vi "GroupOnlyNormalHeavyImplefixaddtimeaddLED.vi"() -> ()   [LabVIEW 2021]
uses:
  ControlforGroupOnlyNormalHeavyImple.ctl
  Control 1.ctl
panel:
  out "speed of train":string
  out "Traffic":string
  out "Traffic condition":string
  out "train":string
  out "Number of Car 2":dbl
  out "Stop of traffic":i32
  out "Wait Time for Train":i32
  out "Number of Car":dbl
  in  "stop":bool
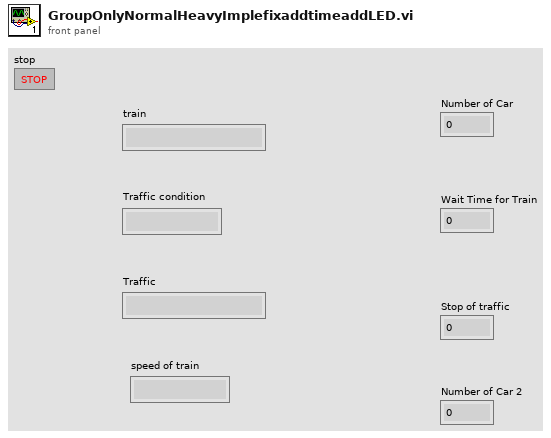
[diagram p1: front panel]
types:
  T1 = typedef "Control 1.ctl" = enum16{"wait", "Down", "Up"}
  T2 = typedef "ControlforGroupOnlyNormalHeavyImple.ctl" = enum16{"Normal", "Heavy", "AfterHeavy"}
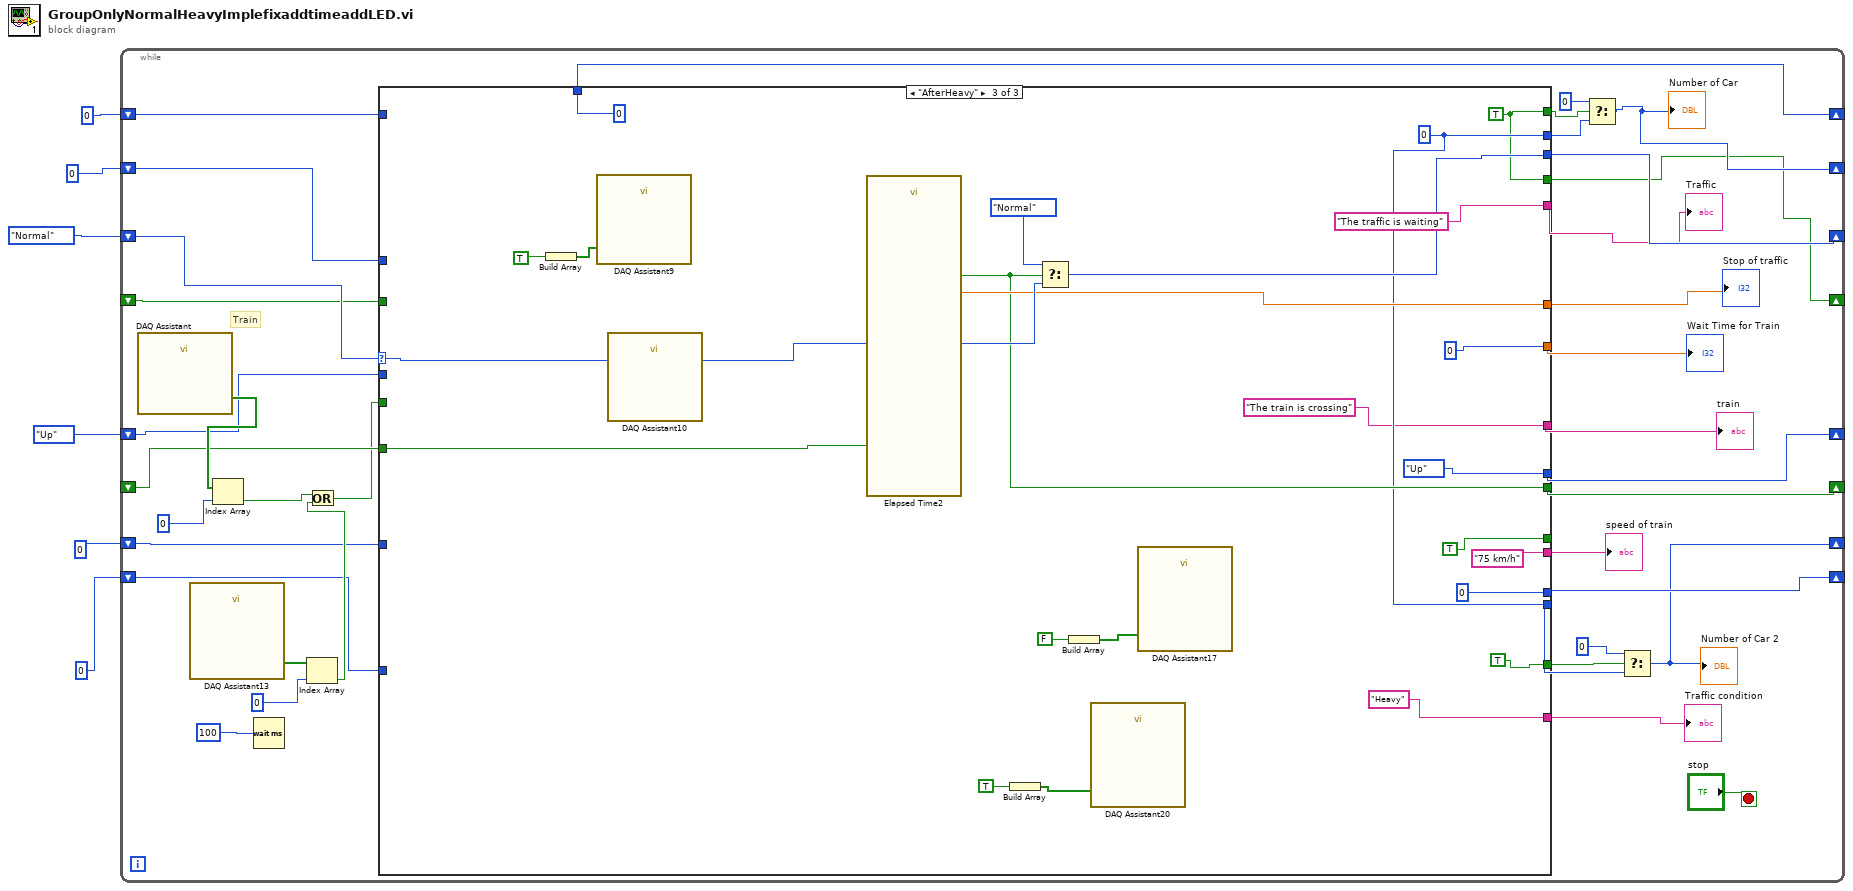
[diagram p0: block diagram]
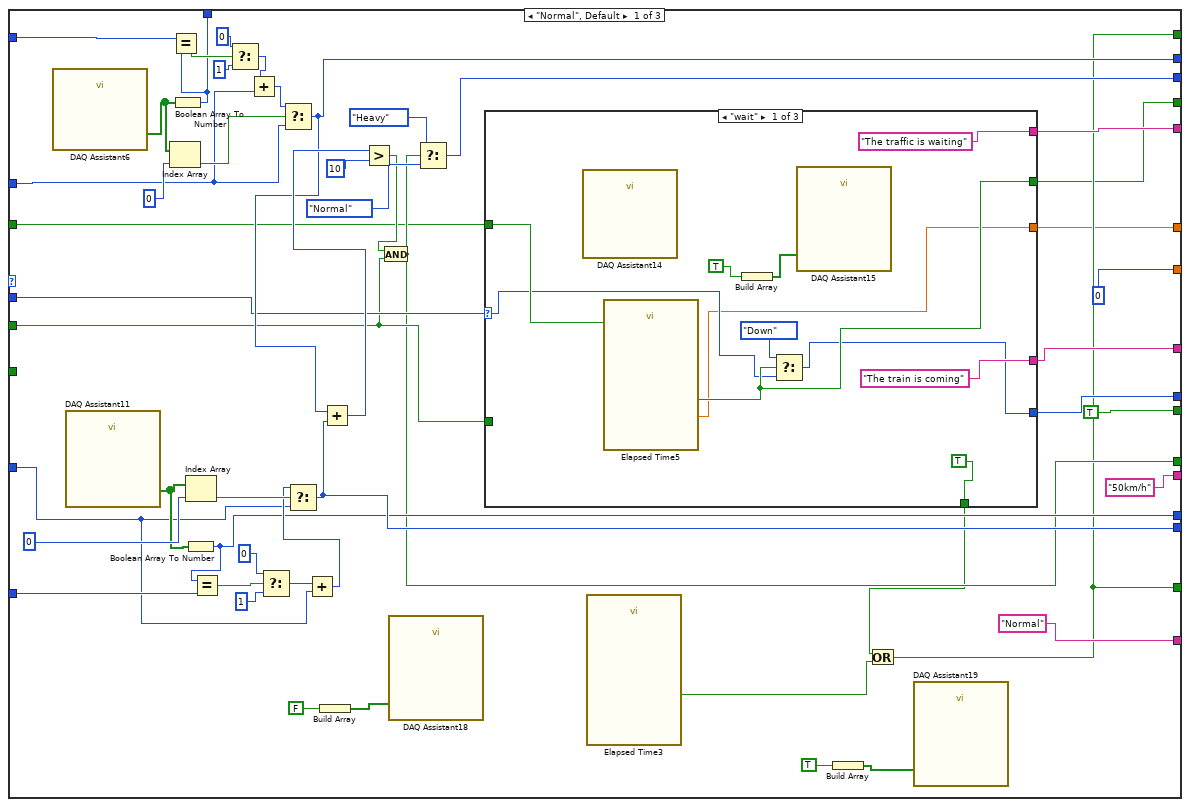
[diagram p2: hidden frame]
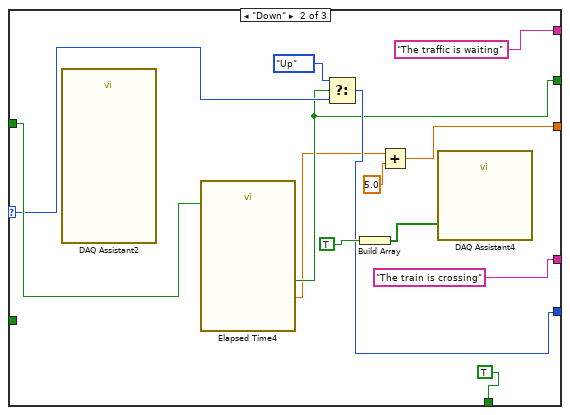
[diagram p3: hidden frame]
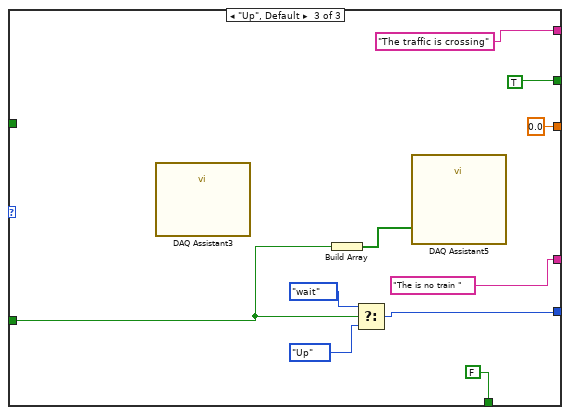
[diagram p4: hidden frame]
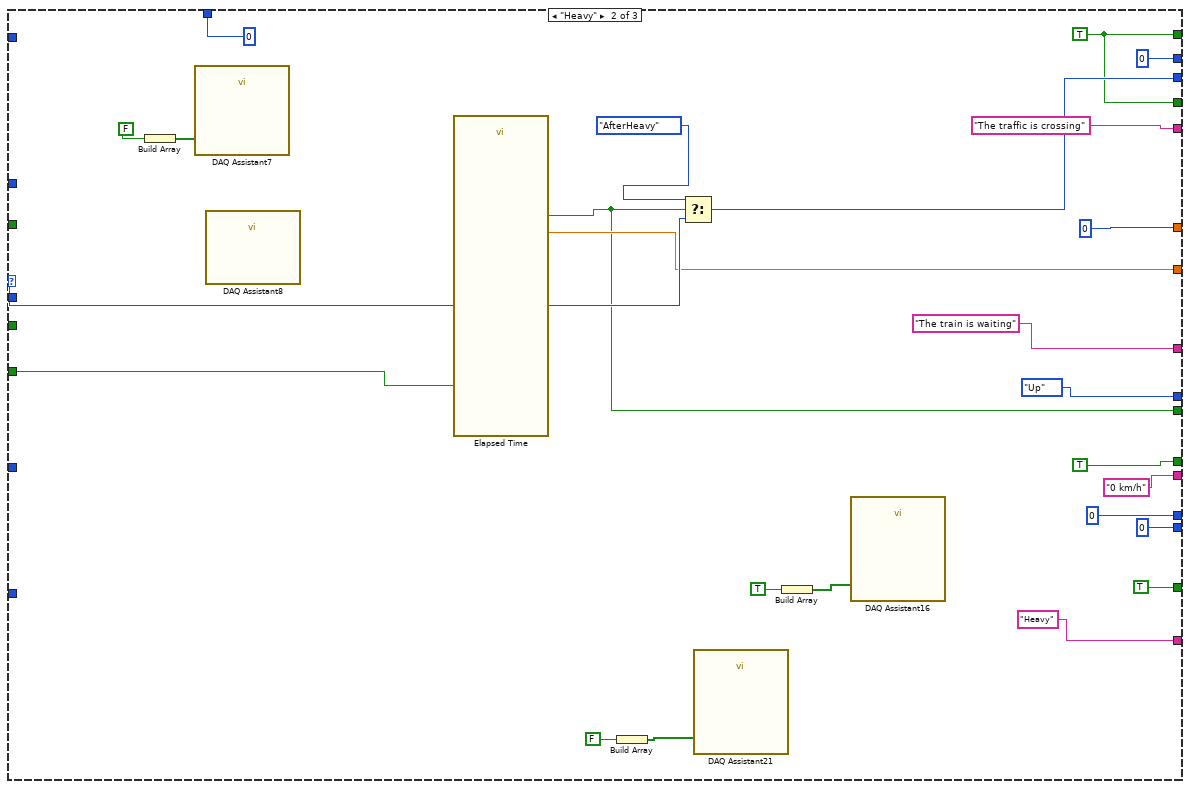
[diagram p5: hidden frame]
diagram:
  n1 = while {
    shift-right: [w41] -> _
    shift-left: ControlforGroupOnlyNormalHeavyImple."Normal" -> [w40]
    shift-right: [w14] -> _
    shift-left: 0 -> [w29]
    shift-right: [w36] -> _
    shift-left: _ -> [w35]
    shift-right: [w18] -> _
    shift-left: 0 -> [w28]
    shift-right: [w16] -> _
    shift-left: 0 ("index") -> [w27]
    shift-right: [w25] -> _
    shift-left: Control_1."Up" -> [w26]
    shift-right: [w23] -> _
    shift-left: 0 ("index") -> [w24]
    shift-right: [w12] -> _
    shift-left: _ -> [w11]
    stop <- "stop" stop-if-true
    # "Train"
    n2 = call "DAQ Assistant"() -> ("data"=w42:bool[])  [unwired: 17 in, 2 out]
    n3 = call "DAQ Assistant13"() -> ("data"=w33:bool[])  [unwired: 17 in, 2 out]
    n4 = Index Array(array=w42, index=0) -> (element=w32:bool)
    n5 = Wait (ms)(milliseconds to wait=100) -> ()  [unwired: 1 out]
    n6 = Index Array(array=w33, index=0) -> (element=w31:bool)
    n7 = Or(x=w32, y=w31) -> (x .or. y?=w21:bool)
    n8 = case shown="\"AfterHeavy\"" w40 {
      selector: w40 -> [_ w148 w173]
      tunnel: w21 -> [w56 _ _]
      tunnel: [w90 w149 w172] -> w41
      tunnel: w29 -> [w69 _ _]
      tunnel: [w84 0 w167] -> w15
      tunnel: [w51 0 w170] -> w38
      tunnel: [0 w146 0] -> w37
      tunnel: [TRUE w145 w169] -> w36
      tunnel: w35 -> [_ w144 w168]
      tunnel: w28 -> [w61 _ _]
      tunnel: [w85 0 w167] -> w19
      tunnel: w27 -> [w82 _ _]
      tunnel: [w77 u32 0 ("index") u32 0 ("index")] -> w16
      tunnel: w26 -> [w76 _ _]
      tunnel: [w75 Control_1."Up" Control_1."Up"] -> w25
      tunnel: w24 -> [w62 _ _]
      tunnel: [w63 u32 0 u32 0] -> w23
      tunnel: ["Normal" "Heavy" "Heavy"] -> w22
      tunnel: [w59 "The train is waiting" "The train is crossing"] -> w9
      tunnel: [w58 "The traffic is crossing" "The traffic is waiting"] -> w10
      tunnel: [w55 TRUE TRUE] -> _
      tunnel: [w52 TRUE TRUE] -> w8
      tunnel: [w52 w131 w156] -> w13
      tunnel: [w50 w131 w156] -> w12
      tunnel: w11 -> [w49 _ _]
      tunnel: ["50km/h" "0 km/h" "75 km/h"] -> w7
      frame "Normal", Default {
        n9 = call "DAQ Assistant6"() -> ("data"=w80:bool[])  [unwired: 17 in, 2 out]
        n10 = call "DAQ Assistant11"() -> ("data"=w74:bool[])  [unwired: 17 in, 2 out]
        n11 = Index Array(array=w80, index=0) -> (element=w81:bool)
        n12 = Boolean Array To Number(Boolean array=w80) -> (number=w77:u32)
        n13 = Equal?(x=w82, y=w77) -> (x = y?=w79:bool)
        n14 = Index Array(array=w74, index=0) -> (element=w65:bool)
        n15 = Boolean Array To Number(Boolean array=w74) -> (number=w63:u32)
        n16 = Equal?(x=w63, y=w62) -> (x = y?=w73:bool)
        n17 = Select(t=0, s=w79, f=1) -> (s? t:f=w70:i32)
        n18 = Add(x=w70, y=w69) -> (x+y=w68:i32)
        n19 = Select(t=0, s=w73, f=1) -> (s? t:f=w66:i32)
        n20 = Select(t=w68, s=w81, f=w69) -> (s? t:f=w84:i32)
        n21 = Add(x=w66, y=w61) -> (x+y=w64:i32)
        n22 = Select(t=w64, s=w65, f=w61) -> (s? t:f=w85:i32)
        n23 = Build Array(FALSE) -> (w48:bool[])
        n24 = Add(x=w84, y=w85) -> (x+y=w86:i32)
        n25 = Greater?(x=w86, y=10) -> (0:w57:bool)
        n26 = And(x=w57, y=w56) -> (x .and. y?=w55:bool)
        n27 = call "DAQ Assistant18"("data"=w48) -> ()  [unwired: 17 in, 2 out]
        n28 = Select(t=ControlforGroupOnlyNormalHeavyImple."Heavy", s=w55, f=ControlforGroupOnlyNormalHeavyImple."Normal") -> (s? t:f=w90:T2)
        n29 = case shown="\"wait\"" w76 {
          selector: w76 -> [w96 w110 _]
          tunnel: w56 -> [_ _ w120]
          tunnel: [w98 w109 w126] -> w75
          tunnel: ["The train is coming" "The train is crossing" "The is no train "] -> w59
          tunnel: ["The traffic is waiting" "The traffic is waiting" "The traffic is crossing"] -> w58
          tunnel: [TRUE TRUE FALSE] -> w53
          tunnel: [w95 w105 0.0 ("Elapsed Time (s)")] -> w51
          tunnel: [w99 w108 TRUE] -> w50
          tunnel: w49 -> [w100 w112 _]
          frame "wait" {
            n30 = call "DAQ Assistant14"() -> ()  [unwired: 18 in, 2 out]
            n31 = call "Elapsed Time5"("Reset"=w100) -> ("Elapsed Time (s)"=w95:dbl, "Time has Elapsed"=w99:bool)  [unwired: 11 in, 6 out]
            n32 = Build Array(TRUE) -> (w104:bool[])
            n33 = Select(t=Control_1."Down", s=w99, f=w96) -> (s? t:f=w98:T1)
            n34 = call "DAQ Assistant15"("data"=w104) -> ()  [unwired: 17 in, 2 out]
          }
          frame "Down" {
            n35 = call "DAQ Assistant2"() -> ()  [unwired: 18 in, 2 out]
            n36 = call "Elapsed Time4"("Reset"=w112) -> ("Elapsed Time (s)"=w106:dbl, "Time has Elapsed"=w108:bool)  [unwired: 11 in, 6 out]
            n37 = Select(t=Control_1."Up", s=w108, f=w110) -> (s? t:f=w109:T1)
            n38 = Build Array(TRUE) -> (w117:bool[])
            n39 = Add(x=w106, y=5.0) -> (x+y=w105:dbl)
            n40 = call "DAQ Assistant4"("data"=w117) -> ()  [unwired: 17 in, 2 out]
          }
          frame "Up", Default {
            n41 = call "DAQ Assistant3"() -> ()  [unwired: 18 in, 2 out]
            n42 = Build Array(w120) -> (w127:bool[])
            n43 = Select(t=Control_1."wait", s=w120, f=Control_1."Up") -> (s? t:f=w126:T1)
            n44 = call "DAQ Assistant5"("data"=w127) -> ()  [unwired: 17 in, 2 out]
          }
        }
        n45 = call "Elapsed Time3"() -> ("Time has Elapsed"=w54:bool)  [unwired: 12 in, 7 out]
        n46 = Build Array(TRUE) -> (w44:bool[])
        n47 = Or(x=w53, y=w54) -> (x .or. y?=w52:bool)
        n48 = call "DAQ Assistant19"("data"=w44) -> ()  [unwired: 17 in, 2 out]
      }
      frame "Heavy" {
        w131 = TRUE
        n49 = Build Array(FALSE) -> (w151:bool[])
        n50 = call "DAQ Assistant7"("data"=w151) -> ()  [unwired: 17 in, 2 out]
        n51 = call "DAQ Assistant8"() -> ()  [unwired: 18 in, 2 out]
        n52 = call "Elapsed Time"("Reset"=w144) -> ("Elapsed Time (s)"=w146:dbl, "Time has Elapsed"=w145:bool)  [unwired: 11 in, 6 out]
        n53 = Build Array(FALSE) -> (w128:bool[])
        n54 = Select(t=ControlforGroupOnlyNormalHeavyImple."AfterHeavy", s=w145, f=w148) -> (s? t:f=w149:T2)
        n55 = call "DAQ Assistant21"("data"=w128) -> ()  [unwired: 17 in, 2 out]
        n56 = Build Array(TRUE) -> (w137:bool[])
        n57 = call "DAQ Assistant16"("data"=w137) -> ()  [unwired: 17 in, 2 out]
      }
      frame "AfterHeavy" {
        w156 = TRUE
        w167 = 0
        n58 = Build Array(TRUE) -> (w175:bool[])
        n59 = call "DAQ Assistant9"("data"=w175) -> ()  [unwired: 17 in, 2 out]
        n60 = call "DAQ Assistant10"() -> ()  [unwired: 18 in, 2 out]
        n61 = call "Elapsed Time2"("Reset"=w168) -> ("Elapsed Time (s)"=w170:dbl, "Time has Elapsed"=w169:bool)  [unwired: 11 in, 6 out]
        n62 = Build Array(TRUE) -> (w154:bool[])
        n63 = Select(t=ControlforGroupOnlyNormalHeavyImple."Normal", s=w169, f=w173) -> (s? t:f=w172:T2)
        n64 = Build Array(FALSE) -> (w161:bool[])
        n65 = call "DAQ Assistant20"("data"=w154) -> ()  [unwired: 17 in, 2 out]
        n66 = call "DAQ Assistant17"("data"=w161) -> ()  [unwired: 17 in, 2 out]
      }
    }
    "Wait Time for Train" <- w37
    "Stop of traffic" <- w38
    "Traffic condition" <- w22
    "train" <- w9
    "Traffic" <- w10
    "speed of train" <- w7
    n67 = Select(t=0, s=w13, f=w15) -> (s? t:f=w14:i32)
    "Number of Car" <- w14
    n68 = Select(t=0, s=w8, f=w19) -> (s? t:f=w18:i32)
    "Number of Car 2" <- w18
  }
